vi "Restore Matrix Property.vi"(6 "Control Ref Queue":T4, 8 "error in (no error)":errorcluster, 10 "Matrix Representation Array In":T1, 11 "2D Plotmatrix.lvclass in":refnum<class "XY Plot Matrix.lvclass">) -> (0 "error out":errorcluster, 2 "Matrix Representation Array Out":T1, 3 "2D Plotmatrix.lvclass out":refnum<class "XY Plot Matrix.lvclass">)   [LabVIEW 2017, in "XY Plot Matrix.lvclass"]
uses:
  <vilib>/Math Plots/2D Math Plots/XY Plot Matrix/XY Plot Matrix/XY Plot Matrix.lvclass
  <vilib>/Math Plots/2D Math Plots/2D Plot/Action String/XYPlotMatrix Ctrl Act Queue.ctl
  <vilib>/Math Plots/2D Math Plots/2D Plot/Action String/XYPlotMatrix Ctrl Act Cluster.ctl
  <vilib>/Math Plots/2D Math Plots/2D Plot/Action String/2DMathPlot State Class.ctl
  e:/builds/penguin/labview/branches/2017/dev/dist/vi.lib/Math Plots/2D Math Plots/2D Plot/2D Plot/2D Plot.lvclass
  <vilib>/Math Plots/2D Math Plots/XY Plot Matrix/XY Plot Matrix/Typedef/Mulitmatrix Representation.ctl
  <vilib>/Math Plots/2D Math Plots/XY Plot Matrix/XY Plot Matrix/Typedef/Matrix Representation.ctl
  <vilib>/Math Plots/2D Math Plots/2D Plot/2D Plot/Typedef/Range Cluster.ctl
  <vilib>/Math Plots/2D Math Plots/2D Plot/2D Plot/2D Plot.lvclass
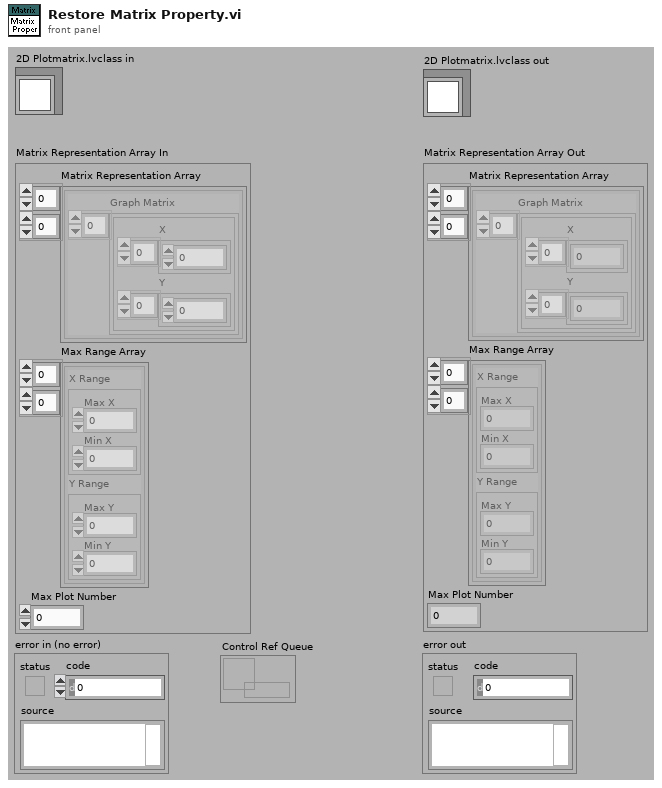
[diagram p1: front panel]
types:
  T1 = typedef "XY Plot Matrix.lvclass/Mulitmatrix Representation.ctl" = cluster{"Matrix Representation Array":T2[][], "Max Range Array":T3[][], "Max Plot Number":i32}
  T2 = typedef "XY Plot Matrix.lvclass/Matrix Representation.ctl" = cluster{"Graph Matrix":cluster{"X":dbl[], "Y":dbl[]}[]}
  T3 = typedef "2D Plot.lvclass/Range Cluster.ctl" = cluster{"X Range":cluster{"Max X":dbl, "Min X":dbl}, "Y Range":cluster{"Max Y":dbl, "Min Y":dbl}}
  T4 = typedef "XYPlotMatrix Ctrl Act Queue.ctl" = refnum<queue>
  T5 = typedef "2DMathPlot State Class.ctl" = enum16{"Update All (Undo)", "Update General", "Update Appearance", "Update Format", "Update Scale", "Update Marker", "Update Cursor", "None"}
  T6 = typedef "XYPlotMatrix Ctrl Act Cluster.ctl" = cluster{"Facade VI":refnum<vi>, "XControl":refnum<vi>, "Sub Panel":refnum<vi>, "Sub VI":refnum<vi>, "Export Image":refnum<vi>, "Display State Change Class":T5}
  T7 = typedef "2D Plot.lvclass/Property Cluster.ctl" = cluster{"Graph General":T8, "Format Property":string[], "Scale Array":T9, "Cursor Property":T12, "Annotation List":T14, "Active Cursor":i32, "Active Plot":i32}
  T8 = typedef "2D Plot.lvclass/Graph General Property.ctl" = cluster{"Palette Visible":cluster{"Graph Legend":bool, "Plot Legend":bool, "Auto size":bool, "Number of Plots":u32, "X Scrollbar":bool, "Scale Legend":bool, "Cursor Legend":bool}, "Plot Area Color":cluster{"FG Color":u32, "BG Color":u32}, "Bounds Size":cluster{"Width":u32, "Height":u32}, "Plot Area Bounds":cluster{"Left":i16, "Top":i16, "Right":i16, "Bottom":i16}}
  T9 = typedef "2D Plot.lvclass/Scale Array.ctl" = T10[]
  T10 = typedef "2D Plot.lvclass/Scale Cluster.ctl" = cluster{"General":cluster{"Editable":bool, "Flipped":bool, "Mapping Mode":u8, "Visible":bool, "Style":u8, "Scale Fit":u8}, "Offset and Multiplier":T11, "Range":cluster{"Minimum":dbl, "Maximum":dbl, "Increment":dbl, "Minor Increment":dbl, "Start":dbl}, "Tick Color":cluster{"Major Color":u32, "Minor Color":u32}, "Gird Color":cluster{"Major Color":u32, "Minor Color":u32}, "Marker":cluster{"Visible":bool, "FG Color":u32, "BG Color":u32, "Font Name":string, "Font Size":u32, "Font Bold":bool, "Font Italic":bool, "Font Strikeout":bool, "Font Underline":bool}, "Name Label":cluster{"Visible":bool, "FG Color":u32, "BG Color":u32, "Font Name":string, "Font Size":u32, "Font Bold":bool, "Font Italic":bool, "Font Strikeout":bool, "Font Underline":bool, "Justification":enum16{"Left", "Center", "Right"}, "Text":string}}
  T11 = typedef "LVOffsetAndMultiplierTypeDef.ctl" = cluster{"Offset":dbl, "Multiplier":dbl}
  T12 = typedef "2D Plot.lvclass/Cursor Property.ctl" = cluster{"Cursor List":T13, "Cursor List Addtional":cluster{"Cursor Selection Color":u32, "Line Style":u8, "Line Width":u8, "Visible":bool}[]}
  T13 = typedef "LVCursorListTypeDef.ctl" = cluster{"Name":string, "Color":u32, "Style":u8, "Point Style":u8, "Name Visible":bool, "Allow Drag":bool, "Cursor Mode":u32, "Plot":i32, "Index":i32, "Position":cluster{"X":dbl, "Y":dbl}, "X Scale":u32, "Y Scale":u32, "Watch Plots":i32[], "Watch All Plots":bool, "Plot Area":i32, "Label Offset":cluster{"X":dbl, "Y":dbl}}[]
  T14 = typedef "LVAnnotationListTypeDef.ctl" = cluster{"Name":string, "Color":u32, "Style":u8, "Point Style":u8, "Name Visible":bool, "Allow Drag":bool, "Annotation Mode":u32, "Plot":i32, "Index":i32, "Position":cluster{"X":dbl, "Y":dbl}, "X Scale":u32, "Y Scale":u32, "Show Arrow":bool, "Lock Name":bool, "Plot Area":i32, "Label Offset":cluster{"X":dbl, "Y":dbl}}[]
  T15 = typedef "LVBoundsTypeDef.ctl" = cluster{"Width":u32, "Height":u32}
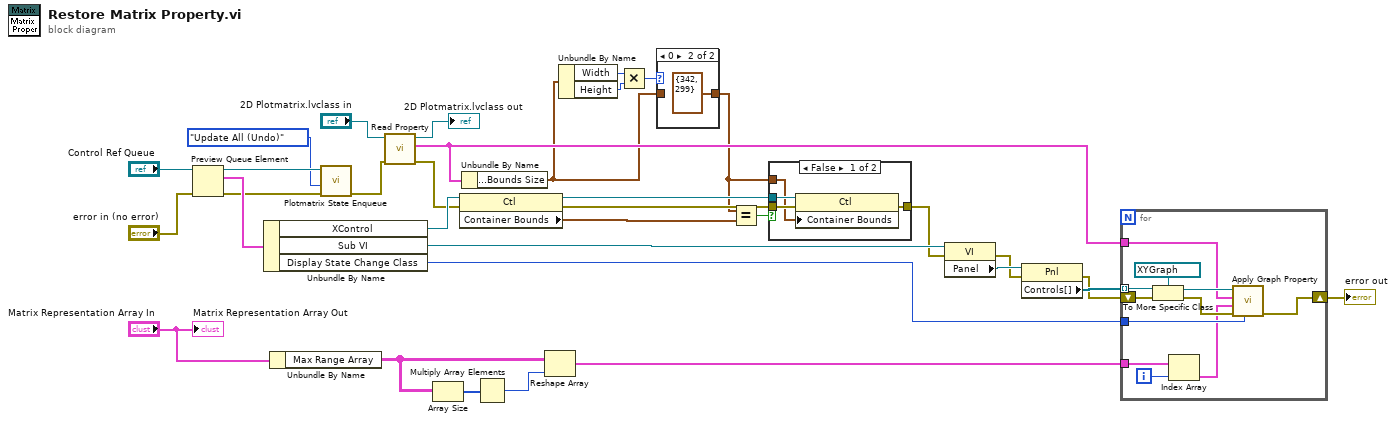
[diagram p0: block diagram]
diagram:
  n1 = Preview Queue Element(queue="Control Ref Queue", error in (no error)="error in (no error)") -> (queue out=w9:T4, element=w31:T6, error out=w10:errorcluster)  [unwired: 2 out]
  n2 = Unbundle By Name(w31) -> ("XControl"=w21:refnum<vi>, "Sub VI"=w32:refnum<vi>, "Display State Change Class"=w11:T5)
  n3 = Unbundle By Name("Matrix Representation Array In") -> ("Max Range Array"=w13:T3[][])
  n4 = call <vilib>:"Plotmatrix State Enqueue.vi"("error in (no error)"=w10, "Display State Change Class"=2DMathPlot_State_Class."Update All (Undo)", "Control Ref Queue"=w9) -> ("error out"=w8:errorcluster)  [unwired: 8 out]
  n5 = call <vilib>:"Read Property.vi"("error in (no error)"=w8, "2D Plot.lvclass in"="2D Plotmatrix.lvclass in") -> ("error out"=w20:errorcluster, "XY Graph Property Cluster"=w23:T7, "2D Plot.lvclass out"=→"2D Plotmatrix.lvclass out":refnum<class "XY Plot Matrix.lvclass">)  [unwired: 7 out]
  n6 = Array Size(array=w13) -> (size(s)=w14:i32[])
  n7 = property class="Ctl"(reference=w21, error in=w20) -> (reference out=w19:refnum<vi>, error out=w18:errorcluster, "Container Bounds"=w17:T15)
  n8 = Unbundle By Name(w23) -> ("Graph General.Bounds Size"=w1:cluster{"Width":u32, "Height":u32})
  n9 = Multiply Array Elements(1:w14) -> (0:w12:i32)
  n10 = Reshape Array(w13, w12) -> (w6:T3[])
  n11 = Unbundle By Name(w1) -> ("Width"=w5:u32, "Height"=w4:u32)
  n12 = Multiply(x=w5, y=w4) -> (x*y=w3:u32)
  n13 = case shown="0" w3 {
    tunnel: [w35 cluster{"Width":u32, "Height":u32} {"Width"=342, "Height"=299} ("Bounds Size")] -> w2
    tunnel: w1 -> [w35 _]
    frame Default {
    }
    frame 0 {
    }
  }
  n14 = Equal?(x=w2, y=w17) -> (x = y?=w16:bool)
  n15 = case shown="False" w16 {
    tunnel: [w40 w41] -> w22
    tunnel: w19 -> [w39 _]
    tunnel: w18 -> [w38 w41]
    tunnel: w2 -> [w37 _]
    frame False {
      n16 = property class="Ctl"(reference=w39, error in=w38, "Container Bounds"=w37) -> (error out=w40:errorcluster)  [unwired: 1 out]
    }
    frame True {
    }
  }
  n17 = property class="VI"(reference=w32, error in=w22) -> (error out=w29:errorcluster, "Panel"=w33:refnum<vi>)  [unwired: 1 out]
  n18 = property class="Pnl"(reference=w33, error in=w29) -> (error out=w28:errorcluster, "Controls[]"=w34:refnum<vi>[])  [unwired: 1 out]
  n19 = for {
    tunnel: w34 -> [w52] mode=indexing
    shift-right: [w46] -> w27
    shift-left: w28 -> [w50]
    tunnel: w23 -> [w47]
    tunnel: w11 -> [w45]
    tunnel: w6 -> [w44]
    i -> [w42]
    n20 = To More Specific Class(target class=refnum<vi> refnum, reference=w52, error in=w50) -> (specific class reference=w49:refnum<vi>, error out=w48:errorcluster)
    n21 = Index Array(array=w44, index=w42) -> (element=w43:T3)
    n22 = call <vilib>:"Apply Graph Property.vi"("Display State Change Class"=w45, "error in (no error)"=w48, "Max Range"=w43, "XY Graph Property Cluster"=w47, "XY Graph"=w49) -> ("error out"=w46:errorcluster)  [unwired: 2 in, 4 out]
  }
  "error out" <- w27
  "Matrix Representation Array Out" <- "Matrix Representation Array In"
